vi "svx_Polar_Read_Attribute.vi"(0 "polar plot":T1, 5 "error in":errorcluster) -> (12 "is OA Polar Plot?":bool, 14 "attribute out":variant, 16 "reference label":u16, 17 "shaft rotating direction":u16, 18 "probe angle [deg]":u16, 19 "error out":errorcluster)   [LabVIEW 2017, in "SVX Polar Plot.xctl"]
uses:
  <vilib>/addons/_XControls/Polar Plot/SVX Polar Plot.xctl
  <vilib>/addons/_NISVFA/_Shared subVIs/Controls/svc_X-Axis Units.ctl
  <vilib>/addons/_XControls/Polar Plot/subVIs/svx_Polar_Attribute.ctl
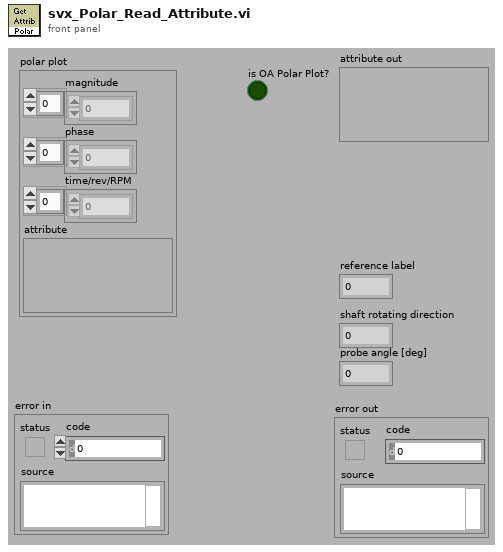
[diagram p1: front panel]
types:
  T1 = cluster{"magnitude":dbl[], "phase":dbl[], "time/rev/RPM":dbl[], "attribute":variant}
  T2 = typedef "SVX Polar Plot.xctl/svx_Polar_Attribute.ctl" = u16
  T3 = typedef "svc_X-Axis Units.ctl" = u16
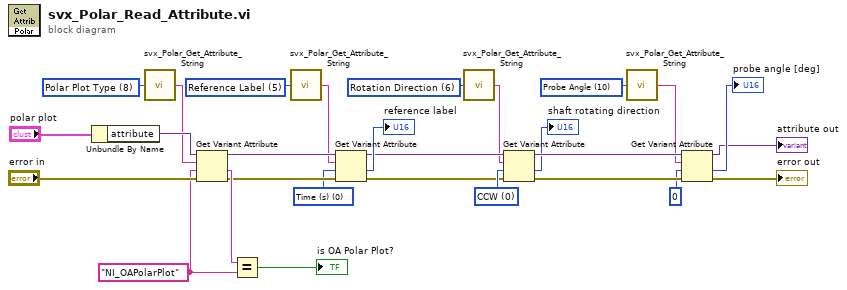
[diagram p0: block diagram]
diagram:
  w2 = T2 10 items=["Pulse / Revolution", "Slope", "Threshold", "Hysteresis", "Order", "Reference Label", "Rotation Direction", "Pair String", "Polar Plot Type", "Sample Per Revolution", "Probe Angle", "Probe Angle X", "Probe Angle Y", "X Axis Unit", "OTB Plot Type"] ("SVMS attribute")
  w4 = T2 6 items=["Pulse / Revolution", "Slope", "Threshold", "Hysteresis", "Order", "Reference Label", "Rotation Direction", "Pair String", "Polar Plot Type", "Sample Per Revolution", "Probe Angle", "Probe Angle X", "Probe Angle Y", "X Axis Unit", "OTB Plot Type"] ("SVMS attribute")
  w6 = T2 5 items=["Pulse / Revolution", "Slope", "Threshold", "Hysteresis", "Order", "Reference Label", "Rotation Direction", "Pair String", "Polar Plot Type", "Sample Per Revolution", "Probe Angle", "Probe Angle X", "Probe Angle Y", "X Axis Unit", "OTB Plot Type"] ("SVMS attribute")
  w8 = T2 8 items=["Pulse / Revolution", "Slope", "Threshold", "Hysteresis", "Order", "Reference Label", "Rotation Direction", "Pair String", "Polar Plot Type", "Sample Per Revolution", "Probe Angle", "Probe Angle X", "Probe Angle Y", "X Axis Unit", "OTB Plot Type"] ("SVMS attribute")
  w9 = T3 0 items=["Time (s)"=0, "Frequency-CB (Hz)"=1, "Frequency-CPB (Hz)"=1248, "Frequency-Arbitrary (Hz)"=2357, "Quefrency (s)"=2, "Revolutions (rev)"=3, "Order"=4, "Speed (RPM)"=11, "Speed (rad/s)"=21, "Index"=65535] ("x-axis units")
  w22 = "NI_OAPolarPlot" ("name")
  w28 = u16 0 items=["CCW", "CW"] ("shaft rotating direction")
  n1 = Unbundle By Name("polar plot") -> ("attribute"=w18:variant)
  n2 = call <vilib>:"svx_Polar_Get_Attribute_String.vi"("SVMS attribute"=w8) -> ("attribute name"=w7:string)  [unwired: 4 in]
  n3 = Get Variant Attribute(Variant=w18, name=w7, default value (empty Variant)=w22, error in="error in") -> (duplicate Variant=w11:variant, value=w23:string, error out=w12:errorcluster)  [unwired: 1 out]
  n4 = Equal?(x=w23, y=w22) -> (x = y?=→"is OA Polar Plot?":bool)
  n5 = call <vilib>:"svx_Polar_Get_Attribute_String.vi"("SVMS attribute"=w6) -> ("attribute name"=w5:string)  [unwired: 4 in]
  n6 = Get Variant Attribute(Variant=w11, name=w5, default value (empty Variant)=w9, error in=w12) -> (duplicate Variant=w14:variant, value=→"reference label":T3, error out=w13:errorcluster)  [unwired: 1 out]
  n7 = call <vilib>:"svx_Polar_Get_Attribute_String.vi"("SVMS attribute"=w4) -> ("attribute name"=w3:string)  [unwired: 4 in]
  n8 = Get Variant Attribute(Variant=w14, name=w3, default value (empty Variant)=w28, error in=w13) -> (duplicate Variant=w27:variant, value=→"shaft rotating direction":u16, error out=w26:errorcluster)  [unwired: 1 out]
  n9 = call <vilib>:"svx_Polar_Get_Attribute_String.vi"("SVMS attribute"=w2) -> ("attribute name"=w1:string)  [unwired: 4 in]
  n10 = Get Variant Attribute(Variant=w27, name=w1, default value (empty Variant)=u16 0 ("probe angle [deg]"), error in=w26) -> (duplicate Variant=→"attribute out":variant, value=→"probe angle [deg]":u16, error out=→"error out":errorcluster)  [unwired: 1 out]
